vi "Get Connection Reference.vi"(8 "error in (no error)":errorcluster, 11 "IP Connection in":refnum<class "IP Connection.lvclass">) -> (0 "error out":errorcluster, 2 "TCP Network Connection":refnum<k5>, 3 "IP Connection out":refnum<class "IP Connection.lvclass">)   [LabVIEW 2011, in "Tinkerforge.lvlib" / "IP Connection.lvclass"]
doc: "This VI returns the connection reference of the IP Connection."
uses:
  IP Connection.lvclass
  IP Connection.lvclass/IP Connection.ctl
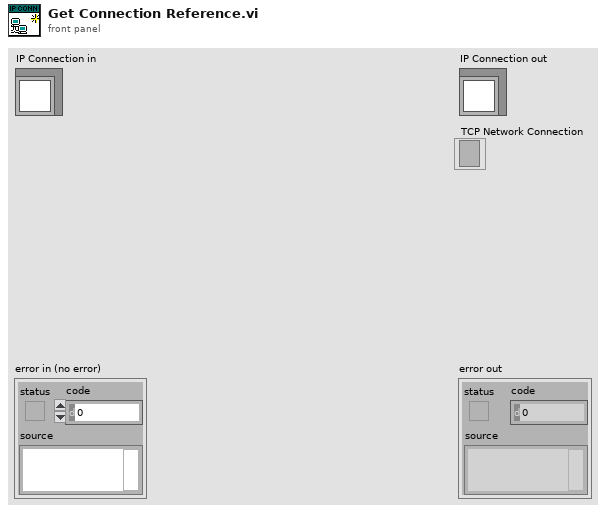
[diagram p1: front panel]
types:
  T1 = typedef "Tinkerforge.lvlib/IP Connection.lvclass/Connection.ctl" = cluster{"TCP Network Connection":refnum<k5>, "is connected":bool, "Connection Status":T2}
  T2 = typedef "Tinkerforge.lvlib/IP Connection.lvclass/Connection Status.ctl" = enum16{"Uninitialized", "Connected", "Reconnecting", "Disconnected"}
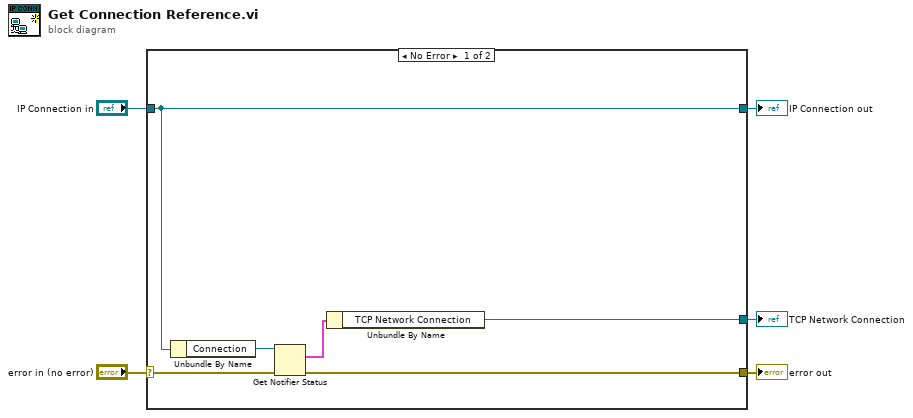
[diagram p0: block diagram]
diagram:
  n1 = case shown="No Error" "error in (no error)" {
    selector: "error in (no error)" -> [w9 w13]
    tunnel: [w8 w13] -> w4
    tunnel: [w11 w12] -> w2
    tunnel: "IP Connection in" -> [w11 w12]
    tunnel: [w6 _] -> w1
    frame No Error {
      n2 = Unbundle By Name(w11) -> ("Connection"=w10:refnum<notifier>)
      n3 = Get Notifier Status(notifier=w10, error in (no error)=w9) -> (current notification=w7:T1, error out=w8:errorcluster)  [unwired: 3 out]
      n4 = Unbundle By Name(w7) -> ("TCP Network Connection"=w6:refnum<k5>)
    }
    frame Error {
    }
  }
  "error out" <- w4
  "IP Connection out" <- w2
  "TCP Network Connection" <- w1
